vi "FileLengthCalc.vi"(1 "StrIn":string) -> (0 "FileLen":u32)   [LabVIEW 2013]
panel:
  out "无符号字节数组":u8[](array[numeric])
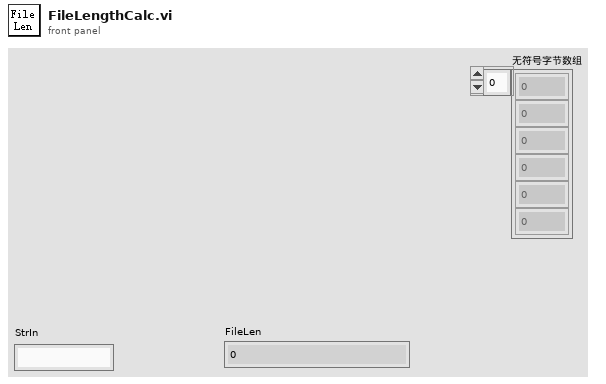
[diagram p1: front panel]
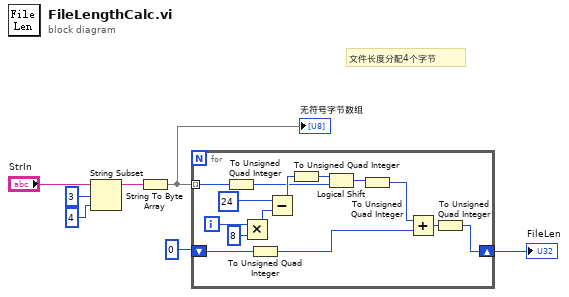
[diagram p0: block diagram]
diagram:
  # "文件长度分配4个字节"
  n1 = String Subset(string="StrIn", offset (0)=3, length (rest)=4) -> (substring=w3:string)
  n2 = String To Byte Array(string=w3) -> (unsigned byte array=w7:u8[])
  "无符号字节数组" <- w7
  n3 = for {
    tunnel: w7 -> [w21] mode=indexing
    shift-right: [w12] -> w4
    shift-left: u64 0 -> [w14]
    i -> [w19]
    n4 = To Unsigned Quad Integer(1:w21) -> (0:w9:u64)
    n5 = Multiply(x=w19, y=u64 8) -> (x*y=w17:u64)
    n6 = To Unsigned Quad Integer(1:w14) -> (0:w11:u64)
    n7 = Subtract(x=u64 24, y=w17) -> (x-y=w18:u64)
    n8 = To Unsigned Quad Integer(1:w18) -> (0:w8:u64)
    n9 = Logical Shift(y=w8, x=w9) -> (x << y=w15:u64)
    n10 = To Unsigned Quad Integer(1:w15) -> (0:w10:u64)
    n11 = Add(x=w10, y=w11) -> (x+y=w13:u64)
    n12 = To Unsigned Quad Integer(1:w13) -> (0:w12:u64)
  }
  "FileLen" <- w4
